vi "Read Coords.vi"(8 "error in (no error)":errorcluster, 11 "ListboxDoubleClickMsg in":refnum<class "ListboxDoubleClickMsg.lvclass">) -> (0 "error out":errorcluster, 2 "Coords":T1, 3 "ListboxDoubleClickMsg out":refnum<class "ListboxDoubleClickMsg.lvclass">)   [LabVIEW 2017, in "ActorEvents.lvlib" / "ListboxDoubleClickMsg.lvclass"]
uses:
  <vilib>/gpm_packages/@cs/mva-viewable/Source/ActorEvents/IEventAggregator Messages/ListboxDoubleClickMsg/ListboxDoubleClickMsg.lvclass
  <vilib>/Utility/miscctls.llb/LVPoint32TypeDef.ctl
  <vilib>/gpm_packages/@cs/mva-viewable/Source/ActorEvents/IEventAggregator Messages/ListboxDoubleClickMsg/ListboxDoubleClickMsg.lvclass/ListboxDoubleClickMsg.ctl
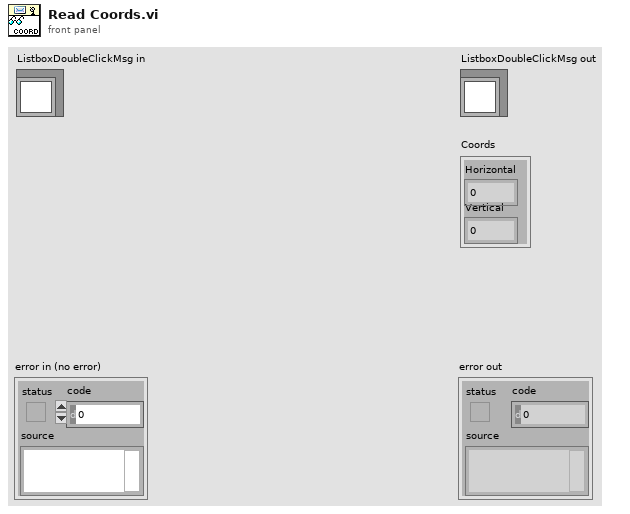
[diagram p1: front panel]
types:
  T1 = typedef "LVPoint32TypeDef.ctl" = cluster{"Horizontal":i32, "Vertical":i32}
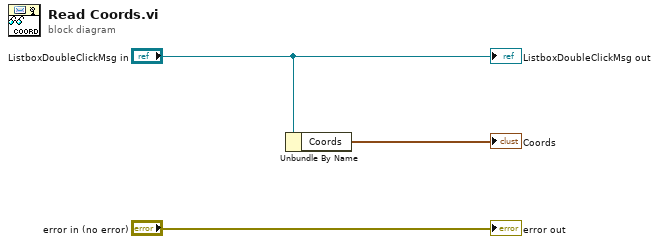
[diagram p0: block diagram]
diagram:
  n1 = Unbundle By Name("ListboxDoubleClickMsg in") -> ("Coords"=→"Coords":T1)
  "error out" <- "error in (no error)"
  "ListboxDoubleClickMsg out" <- "ListboxDoubleClickMsg in"
